vi "FTW-Actor-GetInstanceAddresses.vi"(0 "FTW Actor Instance":refnum<class "FTW-ActorInstance.lvclass">, 11 "error in":errorcluster) -> (4 "FTW Actor Instance out":refnum<class "FTW-ActorInstance.lvclass">, 6 "Inbox Address":string, 15 "error out":errorcluster)   [LabVIEW 2013, in "FTW-ActorInstance.lvclass"]
uses:
  FTW-ActorInstance.lvclass
  FTW-ActorInstance.lvclass/FTW-ActorInstance.ctl
panel:
  # "Inputs"
  # "Outputs"
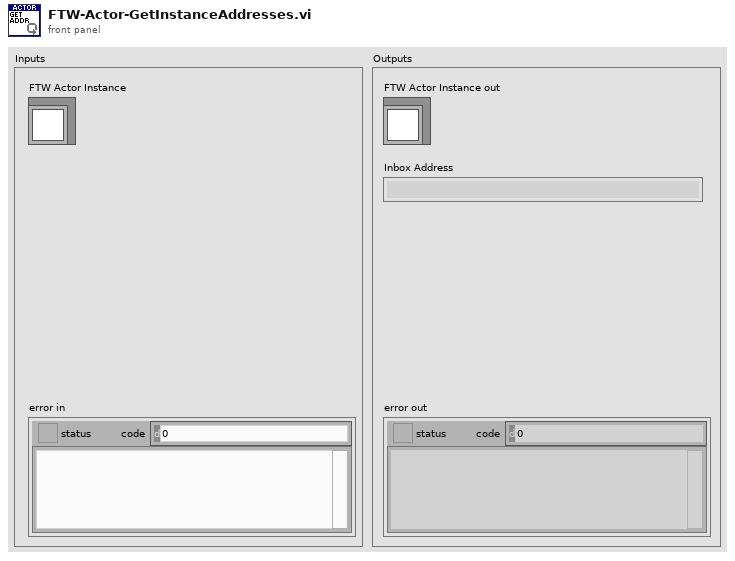
[diagram p1: front panel]
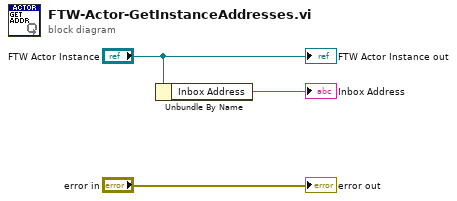
[diagram p0: block diagram]
diagram:
  n1 = Unbundle By Name("FTW Actor Instance") -> ("Inbox Address"=→"Inbox Address":string)
  "FTW Actor Instance out" <- "FTW Actor Instance"
  "error out" <- "error in"
